vi "TCP Chat Window Launcher.vi"() -> ()   [LabVIEW 2020]
uses:
  <vilib>/ni/Actors/Network Endpoint Actors/Protocols/TCP Strategy/TCP Stream Initiator/TCP Stream Initiator.lvclass
  <vilib>/ni/Actors/Network Endpoint Actors/Protocols/TCP Strategy/TCP Stream Listener/TCP Stream Listener.lvclass
  <vilib>/ni/Actors/Network Endpoint Actors/Protocols/TCP Strategy/TCP Stream/TCP Stream.lvclass
  Chat Window/Chat Window.lvclass
  <vilib>/ActorFramework/Actor/Actor.lvclass
panel:
  out "error out":errorcluster
  in  "local port":u16=2001
  in  "Remote Port":u16=2001
  in  "Remote Address":string="127.0.0.1"
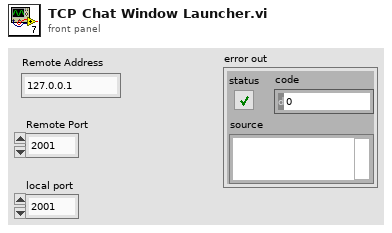
[diagram p1: front panel]
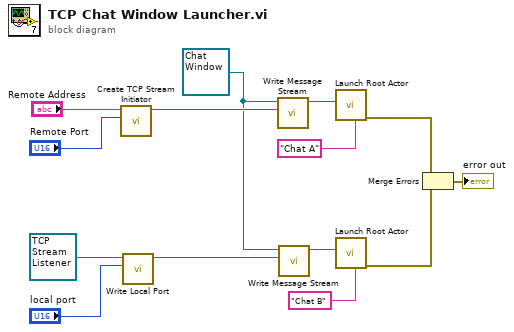
[diagram p0: block diagram]
diagram:
  w9 = refnum<class "Chat Window.lvclass"> refnum ("Chat Window in")
  n1 = call <vilib>:"Create TCP Stream Initiator.vi"("Remote Port"="Remote Port", "Remote Address"="Remote Address") -> ("TCP Stream Initiator"=w10:refnum<class "TCP Stream Initiator.lvclass">)  [unwired: 9 in]
  n2 = call <vilib>:"Write Local Port.vi"("local port"="local port", "TCP Stream in"=refnum<class "TCP Stream Listener.lvclass"> refnum ("TCP Stream Listener.lvclass")) -> ("TCP Stream out"=w1:refnum<class "TCP Stream Listener.lvclass">)  [unwired: 9 in]
  n3 = call "Write Message Stream.vi"("Message Stream"=w10, "Chat Window in"=w9) -> ("Chat Window out"=w8:refnum<class "Chat Window.lvclass">)  [unwired: 9 in]
  n4 = call "Write Message Stream.vi"("Message Stream"=w1, "Chat Window in"=w9) -> ("Chat Window out"=w2:refnum<class "Chat Window.lvclass">)  [unwired: 9 in]
  n5 = call <vilib>:"Launch Root Actor.vi"("Debug Alias"="Chat A", "Actor"=w8) -> ("error out"=w5:errorcluster)  [unwired: 8 in, 1 out]
  n6 = call <vilib>:"Launch Root Actor.vi"("Debug Alias"="Chat B", "Actor"=w2) -> ("error out"=w4:errorcluster)  [unwired: 8 in, 1 out]
  n7 = Merge Errors(w5, w4) -> (→"error out":errorcluster)
